vi "populateTelemetryElevationData.vi"(8 "error in (no error)":errorcluster, 11 "Model in":refnum<class "Model.lvclass">) -> (0 "error out":errorcluster, 3 "Model out":refnum<class "Model.lvclass">)   [LabVIEW 2016, in "Model.lvclass"]
uses:
  Model.lvclass
  Model.lvclass/Model.ctl
  Common_RT_T7Inclinometer/T7Inclinometer/T7Inclinometer.lvclass/T7Inclinometer.ctl
  Publisher/Publisher.lvclass/Publisher.ctl
  Publisher/Publisher.lvclass
  Common_RT_T7Inclinometer/T7Inclinometer/T7Inclinometer.lvclass
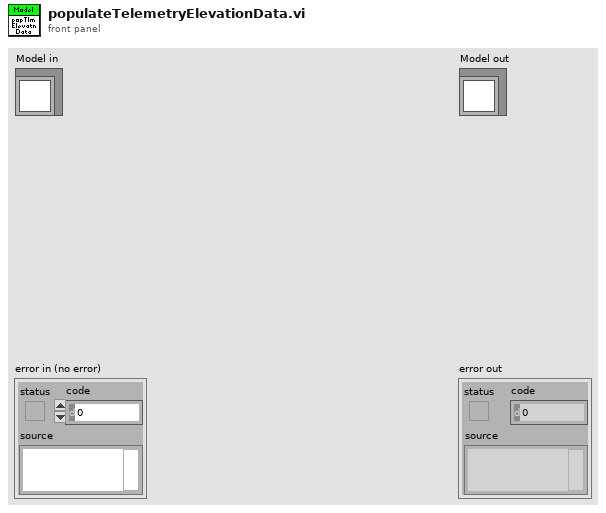
[diagram p1: front panel]
types:
  T1 = typedef "RTT7Inclinometer.lvlib/T7InclinometerData.ctl" = cluster{"Constants":T2, "Telemetry":T3, "Responses":T4, "Timestamps":T6}
  T2 = typedef "RTT7Inclinometer.lvlib/T7InclinometerConstants.ctl" = cluster{"Address":u8}
  T3 = typedef "RTT7Inclinometer.lvlib/T7InclinometerTelemetry.ctl" = cluster{"Angle":dbl}
  T4 = typedef "RTT7Inclinometer.lvlib/T7InclinometerResponses.ctl" = cluster{"ReadAngle":T5}
  T5 = typedef "RTT7Inclinometer.lvlib/T7InclinometerErrors.ctl" = enum16{"None", "InvalidFunctionCodeError", "InvalidRegisterAddressError", "InvalidCRCError", "UnknownAddressError", "UnknownFunctionError", "InvalidResponseLengthError", "UnknownError"}
  T6 = typedef "RTT7Inclinometer.lvlib/T7InclinometerTimestamps.ctl" = cluster{"ReadAngle":dbl}
  T7 = typedef "M1M3SupportTopics.lvlib/TelemetryElevationData.ctl" = cluster{"Timestamp":T8, "InclinometerElevation":dbl, "MeasuredElevation":dbl}
  T8 = typedef "M1M3SupportTopics.lvlib/Timestamp.ctl" = dbl
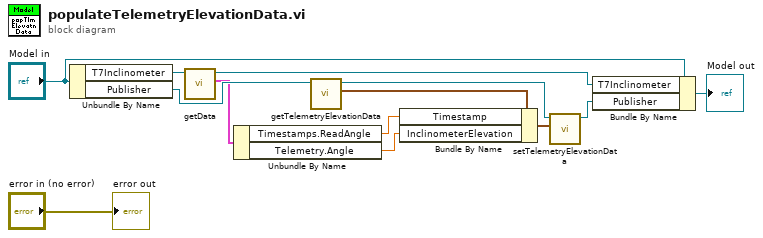
[diagram p0: block diagram]
diagram:
  n1 = Unbundle By Name("Model in") -> ("T7Inclinometer"=w9:refnum<class "T7Inclinometer.lvclass">, "Publisher"=w12:refnum<class "Publisher.lvclass">)
  n2 = call "getData.vi"("T7Inclinometer in"=w9) -> ("T7InclinometerData"=w8:T1, "T7Inclinometer out"=w3:refnum<class "T7Inclinometer.lvclass">)  [unwired: 9 in]
  n3 = Unbundle By Name(w8) -> ("Timestamps.ReadAngle"=w7:dbl, "Telemetry.Angle"=w6:dbl)
  n4 = call "getTelemetryElevationData.vi"("Publisher in"=w12) -> ("TelemetryElevationData"=w11:T7, "Publisher out"=w5:refnum<class "Publisher.lvclass">)  [unwired: 9 in]
  n5 = Bundle By Name(cluster=w11, "Timestamp"=w7, "InclinometerElevation"=w6) -> (w10:T7)
  n6 = call "setTelemetryElevationData.vi"("TelemetryElevationData"=w10, "Publisher in"=w5) -> ("Publisher out"=w4:refnum<class "Publisher.lvclass">)  [unwired: 9 in]
  n7 = Bundle By Name(cluster="Model in", "T7Inclinometer"=w3, "Publisher"=w4) -> (→"Model out":refnum<class "Model.lvclass">)
  "error out" <- "error in (no error)"
